vi "Init Core.vi"(7 "Environment Options (Defaults)":T1, 8 "error in (no error)":errorcluster, 10 "Path Overrides (Empty=Default)":T2 caption="Path Overrides", 11 "WebView2 Control in":refnum<class "WebView2 QControl.lvclass">) -> (0 "error out":errorcluster, 3 "WebView2 Control out":refnum<class "WebView2 QControl.lvclass">)   [LabVIEW 2020, in "WebView2 QControl.lvlib" / "WebView2 QControl.lvclass"]
uses:
  WebView2 QControl.lvclass
  WebView2 QControl.lvclass/WebView2 QControl.ctl
  Webview2 Lib/WebView2 Control Object/WebView2 Control.lvclass
  Paths.ctl
  Core Env Options.ctl
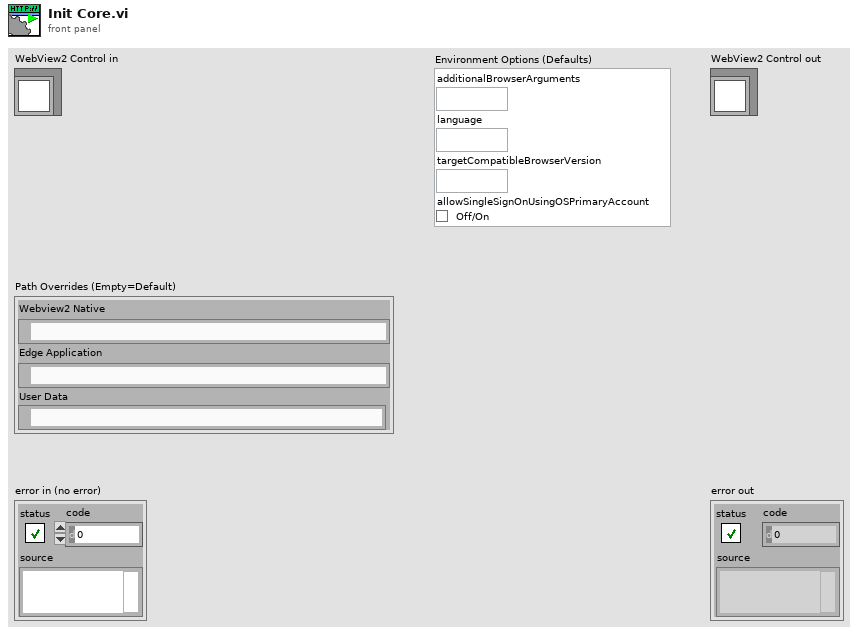
[diagram p1: front panel]
types:
  T1 = typedef "Core Env Options.ctl" = cluster{"additionalBrowserArguments":string, "language":string, "targetCompatibleBrowserVersion":string, "allowSingleSignOnUsingOSPrimaryAccount":bool}
  T2 = typedef "Paths.ctl" = cluster{"Webview2 Native":path, "Edge Application":path, "User Data":path}
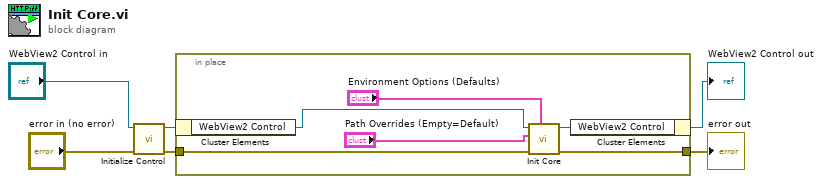
[diagram p0: block diagram]
diagram:
  n1 = call-dynamic "Initialize Control.vi"("error in (no error)"="error in (no error)", "Control in"="WebView2 Control in") -> ("error out"=w1:errorcluster, "Control out"=w3:refnum<class "WebView2 QControl.lvclass">)  [unwired: 8 in]
  n2 = in-place {
    in-place-border: w1 -> [w8]
    in-place-border: [w7] -> w5
    n3 = in-place-cluster #1(w3) -> ("WebView2 Control"=w12:refnum<class "WebView2 Control.lvclass">)
    n4 = call "Init Core.vi"("Environment Options (Defaults)"="Environment Options (Defaults)", "error in (no error)"=w8, "Path Overrides (Empty=Default)"="Path Overrides (Empty=Default)", "WebView2 Control in"=w12) -> ("error out"=w7:errorcluster, "WebView2 Control out"=w11:refnum<class "WebView2 Control.lvclass">)  [unwired: 6 in]
    n5 = in-place-cluster #1("WebView2 Control"=w11) -> (→"WebView2 Control out":refnum<class "WebView2 QControl.lvclass">)
  }
  "error out" <- w5
